vi "Pupulate and conf serial bus.vi"(8 "Error In":errorcluster, 9 "Empty buffer":bool) -> (0 "Error Out":errorcluster, 3 "Devices":refnum<visa-resource-name>[](array[refnum]))   [LabVIEW 2019]
uses:
  <vilib>/Instr/_visa.llb/VISA Find Search Mode.ctl
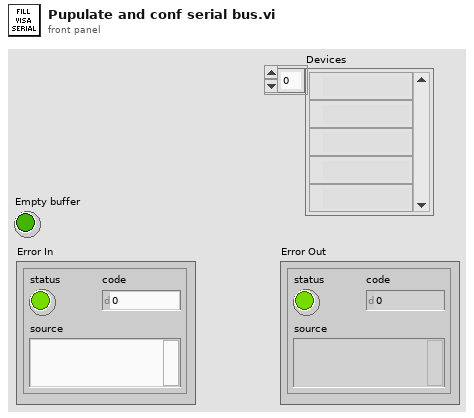
[diagram p1: front panel]
types:
  T1 = typedef "VISA Find Search Mode.ctl" = u32
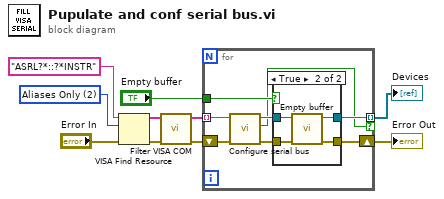
[diagram p0: block diagram]
diagram:
  w10 = T1 2 items=["Canonical Names Only"=0, "Aliases Only"=2, "Include Matching Aliases"=3, "Include All Aliases"=4] ("Search Mode")
  n1 = VISA Find Resource(8:"Error In", 10:w10, 11:"ASRL?*::?*INSTR" ("expression (\"?*\")")) -> (0:w2:errorcluster, 3:w4:string[])  [unwired: 1 out]
  n2 = call "Filter VISA COM.vi"("Error In"=w2, "Names in"=w4) -> ("Error Out"=w1:errorcluster, "COM only list"=w3:string[])  [unwired: 7 in, 1 out]
  n3 = for {
    tunnel: w3 -> [w18] mode=indexing
    tunnel: [w12] -> w8 mode=indexing if=w11
    shift-right: [w14] -> w6
    shift-left: w1 -> [w17]
    tunnel: "Empty buffer" -> [w16]
    n4 = call "Configure serial bus.vi"("Error In"=w17, "VISA resource name"=w18) -> ("Error Out"=w15:errorcluster, "Add instrument"=w11:bool, "VISA resource name 2"=w13:refnum<visa-resource-name>)  [unwired: 7 in]
    n5 = case shown="True" w16 {
      tunnel: w15 -> [w19 w24]
      tunnel: [w19 w23] -> w14
      tunnel: w13 -> [w20 w22]
      tunnel: [w20 w21] -> w12
      frame False {
      }
      frame True {
        n6 = call "Empty buffer.vi"("Error In"=w24, "VISA resource name"=w22) -> ("Error Out"=w23:errorcluster, "VISA resource name out"=w21:refnum<visa-resource-name>)  [unwired: 7 in, 1 out]
      }
    }
  }
  "Devices" <- w8
  "Error Out" <- w6
